vi "Coord window-Insert folder name string.vi"() -> (0 "error out":errorcluster)   [LabVIEW 2020]
uses:
  Globals/Coord window-Globals.vi
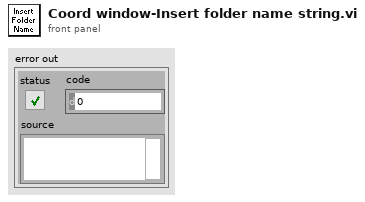
[diagram p1: front panel]
types:
  T1 = typedef "Coordinate list window refs.ctl" = cluster{"Window Name (i.e. Key)":string, "menu reference":refnum<k9>, "VI's reference":refnum<vi>, "Pane 1":refnum<vi>, "Pane 2":refnum<vi>, "Coord Listbox":refnum<vi>, "File name":refnum<vi>, "Picture Map":refnum<vi>, "Stage XYZ Position ind.":refnum<vi>}
  T2 = typedef "LVRowAndColumnTypeDef.ctl" = cluster{"Row":i32, "Column":i32}
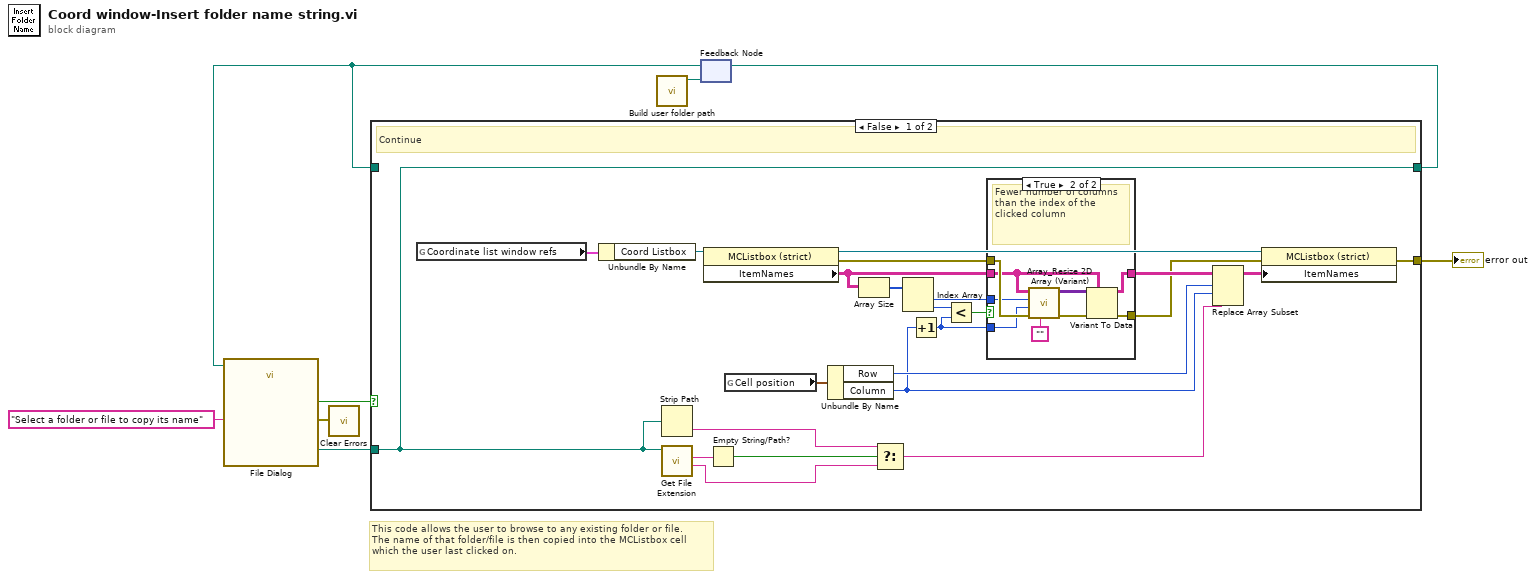
[diagram p0: block diagram]
diagram:
  # "This code allows the user to browse to any existing folder or file.\nThe name of that folder/file is then copied into the MCListbox cell which the user last clicked on."
  n1 = call "Build user folder path.vi"() -> ("Daily folder path with user folder appended?"=w1:path)  [unwired: 11 in]
  n2 = feedback #1(w1) -> (w5:path)
  n3 = call "File Dialog"("start path"=w5, "prompt"="Select a folder or file to copy its name") -> ("selected path"=w7:path, "cancelled"=w6:bool, "error out"=w2:errorcluster)  [unwired: 10 in, 1 out]
  n4 = call <vilib>:"Clear Errors.vi"("error in (no error)"=w2) -> ()  [unwired: 5 in, 2 out]
  n5 = case shown="False" w6 {
    tunnel: [w27 _] -> w8
    tunnel: w7 -> [w21 _]
    tunnel: w5 -> [_ w43]
    tunnel: [w21 w43] -> w4
    frame False {
      # "Continue"
      n6 = global read "Coord window-Globals.vi" "Coordinate list window refs"() -> (w31:T1)
      n7 = Unbundle By Name(w31) -> ("Coord Listbox"=w30:refnum<vi>)
      n8 = Strip Path(path=w21) -> (name=w22:string)  [unwired: 1 out]
      n9 = call <vilib>:"Get File Extension.vi"("file"=w21) -> ("filename without extension"=w23:string, "lowercase file extension"=w25:string)  [unwired: 6 in, 3 out]
      n10 = property class="MCListbox (strict)"(reference=w30) -> (reference out=w28:refnum<vi>, error out=w16:errorcluster, "ItemNames"=w15:string[][])  [unwired: 1 in]
      n11 = Empty String/Path?(string/path=w25) -> (empty?=w24:bool)
      n12 = global read "Coord window-Globals.vi" "Cell position"() -> (w29:T2)
      n13 = Unbundle By Name(w29) -> ("Row"=w20:i32, "Column"=w13:i32)
      n14 = Array Size(array=w15) -> (size(s)=w14:i32[])
      n15 = Select(t=w22, s=w24, f=w23) -> (s? t:f=w19:string)
      n16 = Index Array(array=w14) -> (element #1=w12:i32, element #2=w11:i32)  [unwired: 2 in]
      n17 = Increment(x=w13) -> (x+1=w9:i32)
      n18 = Less?(x=w11, y=w9) -> (x < y?=w10:bool)
      n19 = case shown="True" w10 {
        tunnel: [w33 w40] -> w18
        tunnel: [w32 w39] -> w17
        tunnel: w16 -> [w32 w37]
        tunnel: w15 -> [w33 w36]
        tunnel: w12 -> [_ w35]
        tunnel: w9 -> [_ w34]
        frame False {
        }
        frame True {
          # "Fewer number of columns than the index of the clicked column"
          n20 = call "Array_Resize 2D Array (Variant).vi"("Data type (Array's single element / default values)"="" ("s? t:f"), "Error In"=w37, "Required columns"=w34, "Required rows"=w35, "Array to resize"=w36) -> ("Error Out (no error)"=w38:errorcluster, "Resized array"=w41:variant[][])  [unwired: 5 in]
          n21 = Variant To Data(error in=w38, type=w36, Variant=w41) -> (data=w40:string[][], error out=w39:errorcluster)
        }
      }
      n22 = Replace Array Subset(array=w18, new element=w19, index (row)=w20, index (col)=w13) -> (w26:string[][])
      n23 = property class="MCListbox (strict)"(reference=w28, error in=w17, "ItemNames"=w26) -> (error out=w27:errorcluster)  [unwired: 1 out]
    }
    frame True {
      # "Cancelled"
    }
  }
  "error out" <- w8
  n24 = feedback-in #1(w4) -> ()
